vi "getOpenPort.vi"() -> (0 "port":u16)   [LabVIEW 2013]
doc: "Returns a local port not currently in use."
uses:
  _ROSDefinition.vi
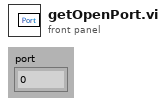
[diagram p1: front panel]
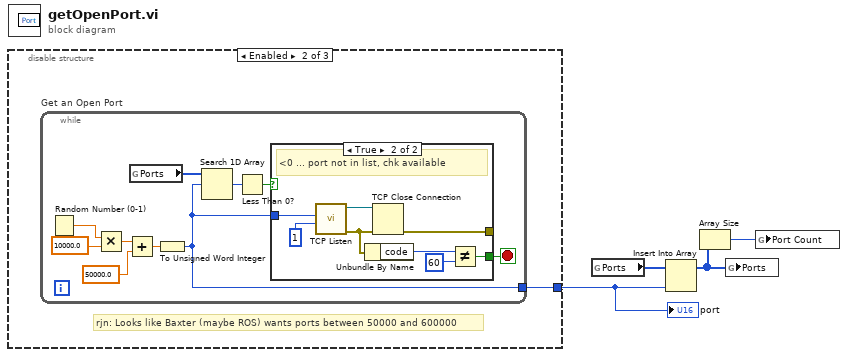
[diagram p0: block diagram]
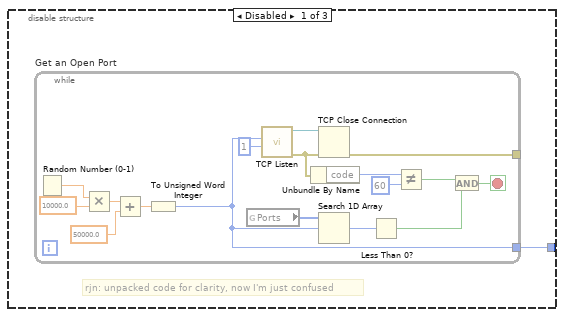
[diagram p2: hidden frame]
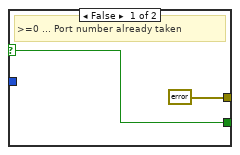
[diagram p3: hidden frame]
diagram:
  n1 = disable-structure shown="Enabled" {
    disable-tunnel: [w5 w23 _] -> w3
    frame Disabled {
      # "rjn: unpacked code for clarity, now I'm just confused"
      n2 = while "Get an Open Port" {
        tunnel: [w10] -> w5
        tunnel: [w12] -> _
        stop <- w8 stop-if-true
        n3 = Random Number (0-1)() -> (number: 0 to 1=w18:dbl)
        n4 = Multiply(x=w18, y=10000.0) -> (x*y=w17:dbl)
        n5 = Add(x=w17, y=50000.0) -> (x+y=w15:dbl)
        n6 = To Unsigned Word Integer(number=w15) -> (unsigned 16bit integer=w10:u16)
        n7 = global read "_ROSDefinition.vi" "Ports"() -> (w11:u16[])
        n8 = call <vilib>:"TCP Listen.vi"("timeout ms (wait forever: -1)"=1, "port"=w10) -> ("error out"=w13:errorcluster, "connection ID"=w14:refnum<k5>)  [unwired: 5 in, 3 out]
        n9 = Unbundle By Name(w13) -> ("code"=w21:i32)
        n10 = TCP Close Connection(connection ID=w14, error in (no error)=w13) -> (error out=w12:errorcluster)  [unwired: 1 in, 1 out]
        n11 = Search 1D Array(1D array=w11, element=w10) -> (index of element=w9:i32)  [unwired: 1 in]
        n12 = Less Than 0?(x=w9) -> (x < 0?=w6:bool)
        n13 = Not Equal?(x=w21, y=60) -> (x != y?=w7:bool)
        n14 = And(x=w7, y=w6) -> (x .and. y?=w8:bool)
      }
    }
    frame Enabled {
      # "rjn: Looks like Baxter (maybe ROS) wants ports between 50000 and 600000"
      n15 = while "Get an Open Port" {
        tunnel: [w27] -> w23
        stop <- w24 stop-if-true
        n16 = Random Number (0-1)() -> (number: 0 to 1=w32:dbl)
        n17 = Multiply(x=w32, y=10000.0) -> (x*y=w31:dbl)
        n18 = Add(x=w31, y=50000.0) -> (x+y=w29:dbl)
        n19 = global read "_ROSDefinition.vi" "Ports"() -> (w28:u16[])
        n20 = To Unsigned Word Integer(number=w29) -> (unsigned 16bit integer=w27:u16)
        n21 = Search 1D Array(1D array=w28, element=w27) -> (index of element=w26:i32)  [unwired: 1 in]
        n22 = Less Than 0?(x=w26) -> (x < 0?=w25:bool)
        n23 = case "If not in list, check if available" shown="True" w25 {
          selector: w25 -> [w34 _]
          tunnel: [errorcluster {"status"=FALSE, "code"=0, "source"=""} ("error out") w38] -> _
          tunnel: w27 -> [_ w37]
          tunnel: [w34 w36] -> w24
          frame False {
            # ">=0 ... Port number already taken"
          }
          frame True {
            # "<0 ... port not in list, chk available"
            n24 = call <vilib>:"TCP Listen.vi"("timeout ms (wait forever: -1)"=1, "port"=w37) -> ("error out"=w39:errorcluster, "connection ID"=w40:refnum<k5>)  [unwired: 5 in, 3 out]
            n25 = Unbundle By Name(w39) -> ("code"=w42:i32)
            n26 = TCP Close Connection(connection ID=w40, error in (no error)=w39) -> (error out=w38:errorcluster)  [unwired: 1 in, 1 out]
            n27 = Not Equal?(x=w42, y=60) -> (x != y?=w36:bool)
          }
        }
      }
    }
    frame Disabled {
    }
  }
  "port" <- w3
  n28 = global read "_ROSDefinition.vi" "Ports"() -> (w4:u16[])
  n29 = Insert Into Array(array=w4, new element=w3) -> (w2:u16[])  [unwired: 1 in]
  n30 = Array Size(array=w2) -> (size(s)=w1:i32)
  n31 = global write "_ROSDefinition.vi" "Ports"(w2) -> ()
  n32 = global write "_ROSDefinition.vi" "Port Count"(w1) -> ()
